vi "Read Encoders.vi"() -> (2 "Right Encoder":dbl, 3 "Left Encoder":dbl)   [LabVIEW 2016]
doc: "Reads encoder inputs"
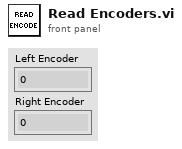
[diagram p1: front panel]
types:
  T1 = typedef "WPI_EncoderDevRef.ctl" = cluster{"DevStatus":errorcluster, "EncoderIndex":T2, "CounterIndex":T3, "DistancePerCount":dbl, "Decoding Type":T4}
  T2 = typedef "FPGA_EncoderIdx.ctl" = enum8{"Enc 0", "Enc 1", "Enc 2", "Enc 3", "Enc 4", "Enc 5", "Enc 6", "Enc 7", "Invalid"}
  T3 = typedef "FPGA_CounterCtrSystemIndex.ctl" = enum8{"Ctr 0", "Ctr 1", "Ctr 2", "Ctr 3", "Ctr 4", "Ctr 5", "Ctr 6", "Ctr 7", "Invalid"}
  T4 = typedef "WPI_EncoderType.ctl" = enum16{"1x", "2x", "4x"}
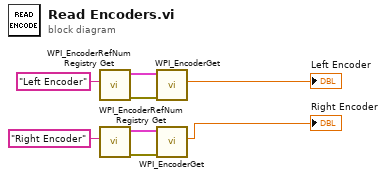
[diagram p0: block diagram]
diagram:
  n1 = call <vilib>:"WPI_EncoderRefNum Registry Get.vi"("refnum name"="Left Encoder") -> ("error out"=w8:errorcluster, "EncoderDevRef"=w7:T1)  [unwired: 9 in]
  n2 = call <vilib>:"WPI_EncoderRefNum Registry Get.vi"("refnum name"="Right Encoder") -> ("error out"=w3:errorcluster, "EncoderDevRef"=w4:T1)  [unwired: 9 in]
  n3 = call <vilib>:"WPI_EncoderGet.vi"("error in (no error)"=w8, "EncoderDevRef"=w7) -> ("Distance"=→"Left Encoder":dbl)  [unwired: 4 in, 5 out]
  n4 = call <vilib>:"WPI_EncoderGet.vi"("error in (no error)"=w3, "EncoderDevRef"=w4) -> ("Distance"=→"Right Encoder":dbl)  [unwired: 4 in, 5 out]
